vi "User Interface.vi"(8 "error in (no error)":errorcluster, 11 "User Interface in":refnum<class "User Interface.lvclass">) -> (0 "error out":errorcluster, 3 "User Interface out":refnum<class "User Interface.lvclass">)   [LabVIEW 2023, in "UDPlog.lvlib" / "UDPlog Transfer Rx User Interface.lvclass"]
uses:
  UDPlog Transfer Rx User Interface.lvclass
  Users/Public/Documents/National Instruments/NI VeriStand 2023/Custom Devices/Data Sharing Framework/Linux_x64/DSF Core.lvlibp/Classes/User Interface/User Interface.lvclass
  Configurations/Rx Transfer/UDPlog Transfer Rx Configuration.lvclass
  C:/Users/Public/Documents/National Instruments/NI VeriStand 2023/Custom Devices/Data Sharing Framework/Linux_x64/DSF Core.lvlibp/Classes/Configuration/Configuration.lvclass
  Configurations/Rx Transfer/UDPlog Transfer Rx Configuration.lvclass/UDPlog Transfer Rx Configuration.ctl
panel:
  in  "Source Address":string
  in  "Source Port":u16
  # "UDP Log UI"
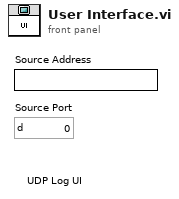
[diagram p1: front panel]
types:
  T1 = typedef "Rx Transfer Settings.ctl" = cluster{"address":u32, "port":u16}
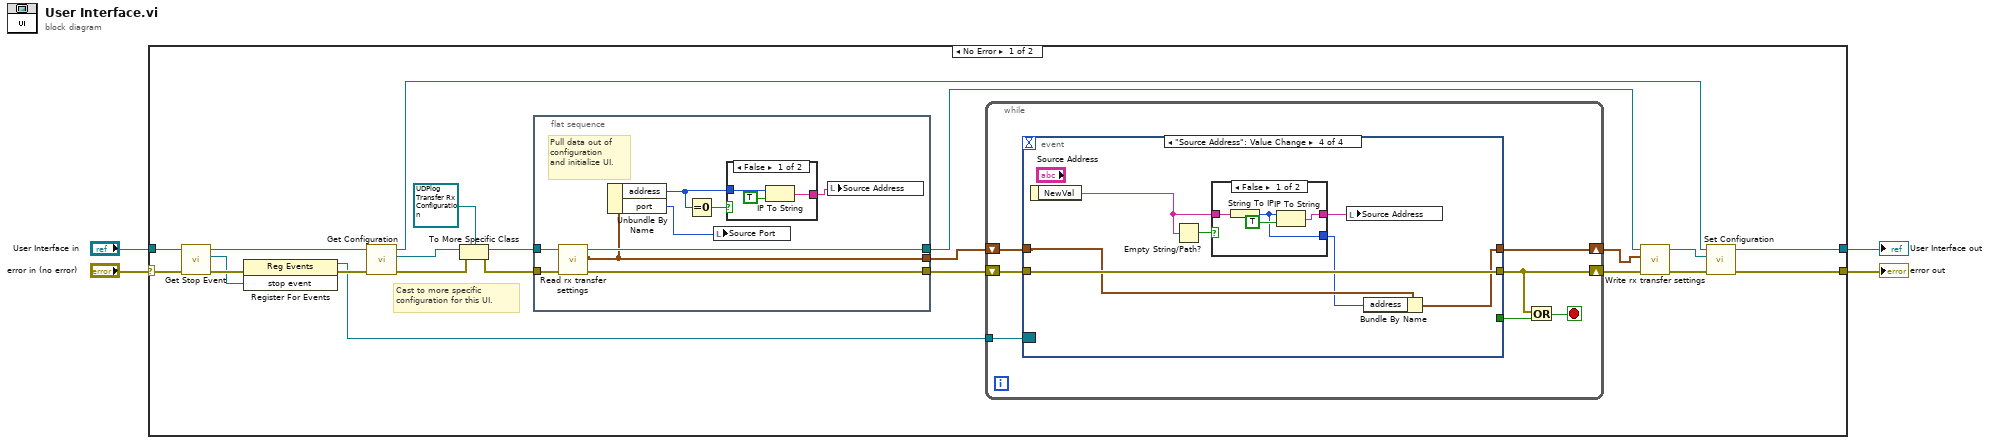
[diagram p0: block diagram]
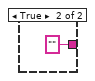
[diagram p2: hidden frame]
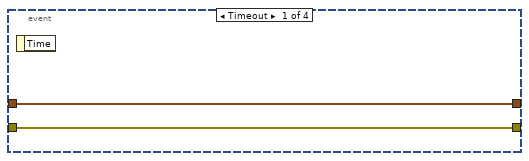
[diagram p3: hidden frame]
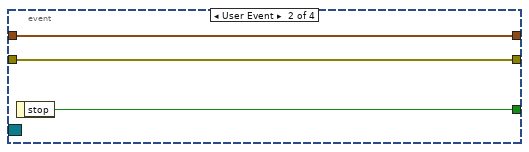
[diagram p4: hidden frame]
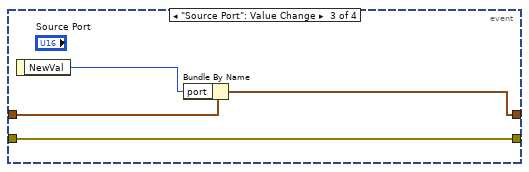
[diagram p5: hidden frame]
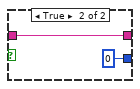
[diagram p6: hidden frame]
diagram:
  n1 = case shown="No Error" "error in (no error)" {
    selector: "error in (no error)" -> [w23 w70]
    tunnel: [w14 w70] -> w4
    tunnel: "User Interface in" -> [w22 w69]
    tunnel: [w13 w69] -> w1
    frame No Error {
      # "Cast to more specific configuration for this UI."
      n2 = call "Get Stop Event.vi"("error in (no error)"=w23, "User Interface in"=w22) -> ("error out"=w21:errorcluster, "stop event"=w20:refnum<user-event>, "User Interface out"=w19:refnum<class "User Interface.lvclass">)  [unwired: 7 in]
      n3 = register-events(error in=w21, w20) -> (reference out=w17:refnum<event-registration>, error out=w18:errorcluster)  [unwired: 1 in]
      n4 = call "Get Configuration.vi"("error in (no error)"=w18, "User Interface in"=w19) -> ("error out"=w16:errorcluster, "configuration"=w15:refnum<class "Configuration.lvclass">, "User Interface out"=w12:refnum<class "User Interface.lvclass">)  [unwired: 7 in]
      n5 = To More Specific Class(target class=refnum<class "UDPlog Transfer Rx Configuration.lvclass"> refnum ("UDPlog.lvlib:UDPlog Transfer Rx Configuration.lvclass"), reference=w15, error in=w16) -> (specific class reference=w26:refnum<class "UDPlog Transfer Rx Configuration.lvclass">, error out=w24:errorcluster)
      n6 = flat-sequence {
        tunnel: [w32] -> w25
        tunnel: w24 -> [w33]
        tunnel: w26 -> [w35]
        tunnel: [w34] -> w6
        tunnel: [w31] -> w7
        frame #0 {
          # "Pull data out of configuration and initialize UI."
          n7 = call "Read rx transfer settings.vi"("error in (no error)"=w33, "UDPlog Transfer Rx Configuration in"=w35) -> ("error out"=w32:errorcluster, "rx transfer settings"=w31:T1, "UDPlog Transfer Rx Configuration out"=w34:refnum<class "UDPlog Transfer Rx Configuration.lvclass">)  [unwired: 7 in]
          n8 = Unbundle By Name(w31) -> ("address"=w29:u32, "port"=w28:u16)
          n9 = Equal To 0?(x=w29) -> (x = 0?=w30:bool)
          n10 = local write "Source Port"(w28) -> ()
          n11 = case shown="False" w30 {
            tunnel: [w38 "" ("name")] -> w27
            tunnel: w29 -> [w37 _]
            frame False {
              n12 = IP To String(1:TRUE ("dot notation? (F)"), 2:w37) -> (0:w38:string)
            }
            frame True {
            }
          }
          n13 = local write "Source Address"(w27) -> ()
        }
      }
      n14 = while {
        tunnel: w17 -> [w46]
        shift-right: [w44] -> w10
        shift-left: w25 -> [w45]
        shift-right: [w40] -> w5
        shift-left: w7 -> [w41]
        stop <- w43 stop-if-true
        n15 = event shown="[3] \"Source Address\": Value Change" {
          selector: w46 -> [_ _ _ _]
          dyn-events: _ -> [_ _ _ _]
          timeout: _ -> [_ _ _ _]
          tunnel: [_ w50 _ _] -> w42
          tunnel: w45 -> [w48 w51 w53 w62]
          tunnel: [w48 w51 w53 w62] -> w44
          tunnel: w41 -> [w47 w49 w55 w58]
          tunnel: [w47 w49 w54 w56] -> w40
          event Timeout {
            n16 = event-data() -> ()  [unwired: 1 in, 1 out]
          }
          event User Event {
            n17 = event-data() -> ("stop"=w50:bool)  [unwired: 1 in]
          }
          event "Source Port": Value Change {
            n18 = event-data() -> ("NewVal"=w52:u16)  [unwired: 1 in]
            n19 = Bundle By Name(cluster=w55, "port"=w52) -> (w54:T1)
          }
          event "Source Address": Value Change {
            n20 = event-data() -> ("NewVal"=w60:string)  [unwired: 1 in]
            n21 = Empty String/Path?(string/path=w60) -> (empty?=w61:bool)
            n22 = case shown="False" w61 {
              tunnel: [w66 w67] -> w59
              tunnel: w60 -> [w65 w67]
              tunnel: [w63 u32 0] -> w57
              frame False {
                n23 = String To IP(1:w65) -> (0:w63:u32)
                n24 = IP To String(1:TRUE ("dot notation? (F)"), 2:w63) -> (0:w66:string)
              }
              frame True {
              }
            }
            n25 = local write "Source Address"(w59) -> ()
            n26 = Bundle By Name(cluster=w58, "address"=w57) -> (w56:T1)
          }
        }
        n27 = Or(x=w44, y=w42) -> (x .or. y?=w43:bool)
      }
      n28 = call "Write rx transfer settings.vi"("error in (no error)"=w10, "rx transfer settings"=w5, "UDPlog Transfer Rx Configuration in"=w6) -> ("error out"=w9:errorcluster, "UDPlog Transfer Rx Configuration out"=w8:refnum<class "UDPlog Transfer Rx Configuration.lvclass">)  [unwired: 7 in]
      n29 = call "Set Configuration.vi"("error in (no error)"=w9, "configuration"=w8, "User Interface in"=w12) -> ("error out"=w14:errorcluster, "User Interface out"=w13:refnum<class "User Interface.lvclass">)  [unwired: 7 in]
    }
    frame Error {
    }
  }
  "error out" <- w4
  "User Interface out" <- w1
